vi "Colour Image to Numpy Array.vi"(8 "error in (no error)":errorcluster, 11 "Refnum in":T1) -> (0 "error out":errorcluster, 3 "Array":u8[][][](array[numeric]))   [LabVIEW 2022 SP3, in "Coin Analyser.lvclass"]
doc: "OpenCV can take an image as a 3d numpy array.\n\nThis converts a colour image to that format - with 3 dimensions for each colour plane."
uses:
  <vilib>/vision/Image Controls.llb/IMAQ Image.ctl
  Coin Analyser.lvclass
  Coin Analyser.lvclass/Coin Analyser.ctl
  <vilib>/vision/NI_Vision_Development_Module.lvlib
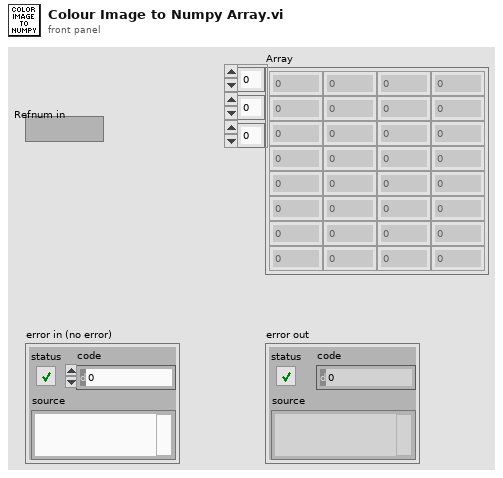
[diagram p1: front panel]
types:
  T1 = typedef "IMAQ Image.ctl" = refnum<image>
  T2 = cluster{"Red (or Hue) value":u8, "Green (or Sat) value":u8, "Blue (or Light or Val) value":u8}[][]
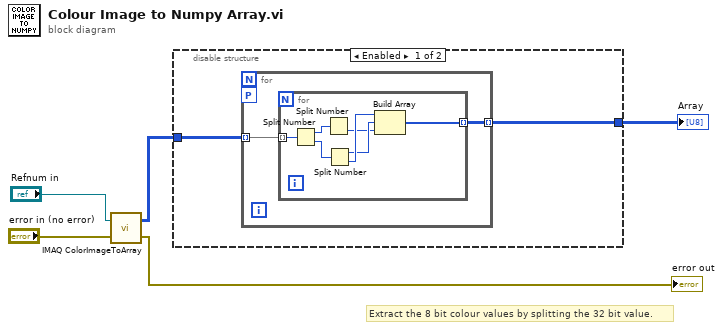
[diagram p0: block diagram]
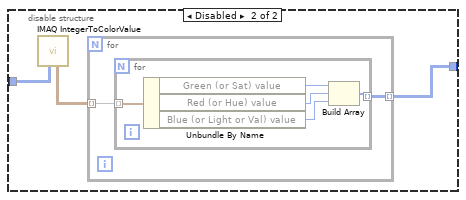
[diagram p2: hidden frame]
diagram:
  # "Extract the 8 bit colour values by splitting the 32 bit value."
  n1 = call "IMAQ ColorImageToArray"("Image"="Refnum in", "error in (no error)"="error in (no error)") -> ("Image Pixels (U32)"=w2:u32[][], "error out"=→"error out":errorcluster)  [unwired: 2 in, 1 out]
  n2 = disable-structure shown="Enabled" {
    disable-tunnel: w2 -> [w7 w19]
    disable-tunnel: [w6 w17] -> w1
    frame Enabled {
      n3 = for {
        tunnel: w7 -> [w9] mode=indexing
        tunnel: [w8] -> w6 mode=indexing
        workers-P: _ -> [_]
        n4 = for {
          tunnel: w9 -> [w16] mode=indexing
          tunnel: [w13] -> w8 mode=indexing
          n5 = Split Number(x=w16) -> (hi(x)=w15:u16, lo(x)=w14:u16)
          n6 = Split Number(x=w15) -> (lo(x)=w10:u8)  [unwired: 1 out]
          n7 = Split Number(x=w14) -> (hi(x)=w11:u8, lo(x)=w12:u8)
          n8 = Build Array(w12, w11, w10) -> (w13:u8[])
        }
      }
    }
    frame Disabled {
      n9 = call "IMAQ IntegerToColorValue"("2D U32 array"=w19) -> ("2D Color value array"=w18:T2)  [unwired: 4 in, 3 out]
      n10 = for {
        tunnel: w18 -> [w21] mode=indexing
        tunnel: [w20] -> w17 mode=indexing
        n11 = for {
          tunnel: w21 -> [w26] mode=indexing
          tunnel: [w22] -> w20 mode=indexing
          n12 = Unbundle By Name(w26) -> ("Green (or Sat) value"=w25:u8, "Red (or Hue) value"=w23:u8, "Blue (or Light or Val) value"=w24:u8)
          n13 = Build Array(w25, w23, w24) -> (w22:u8[])
        }
      }
    }
  }
  "Array" <- w1
